vi "Get Column DBL.vi"(8 "error in (no error)":errorcluster, 11 "PQ Result  in":refnum<class "PQ Result.lvclass">) -> (0 "error out":errorcluster, 2 "DBL":dbl, 3 "PQ Result  out":refnum<class "PQ Result.lvclass">)   [LabVIEW 2015, in "PQ Result.lvclass"]
uses:
  PQ Result.lvclass
  PQ Result.lvclass/PQ Result.ctl
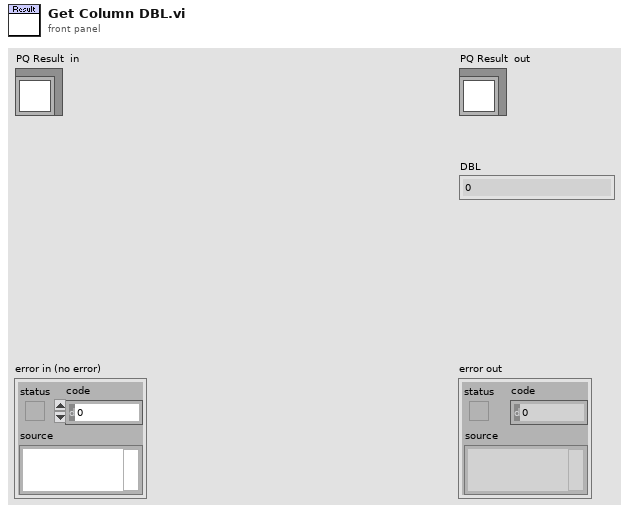
[diagram p1: front panel]
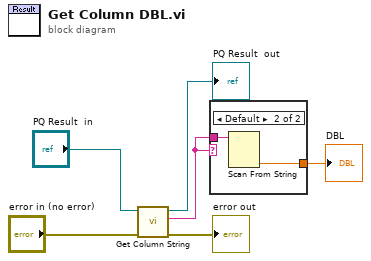
[diagram p0: block diagram]
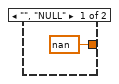
[diagram p2: hidden frame]
diagram:
  n1 = call "Get Column String.vi"("error in (no error)"="error in (no error)", "PQ Result  in"="PQ Result  in") -> ("error out"=→"error out":errorcluster, "String"=w1:string, "PQ Result  out"=→"PQ Result  out":refnum<class "PQ Result.lvclass">)  [unwired: 7 in]
  n2 = case shown="Default" w1 {
    tunnel: w1 -> [_ w9]
    tunnel: [nan w8] -> w2
    frame "", "NULL" {
    }
    frame Default {
      n3 = Scan From String(input string=w9) -> (output 1=w8:dbl)  [unwired: 4 in, 3 out]
    }
  }
  "DBL" <- w2
